vi "BRig_Host__Loop_Producer__UploadLaserParameters_main.vi"() -> ()   [LabVIEW 2014]
uses:
  <vilib>/WebDAVClient/NI_WebDAV.lvlib
panel:
  out "error out":errorcluster
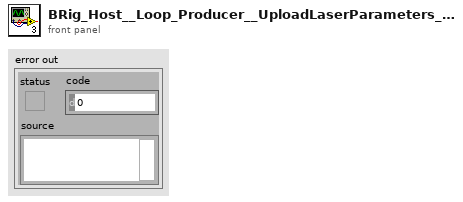
[diagram p1: front panel]
types:
  T1 = typedef "NI_WebDAV.lvlib/SessionHandle.ctl" = refnum<k1>
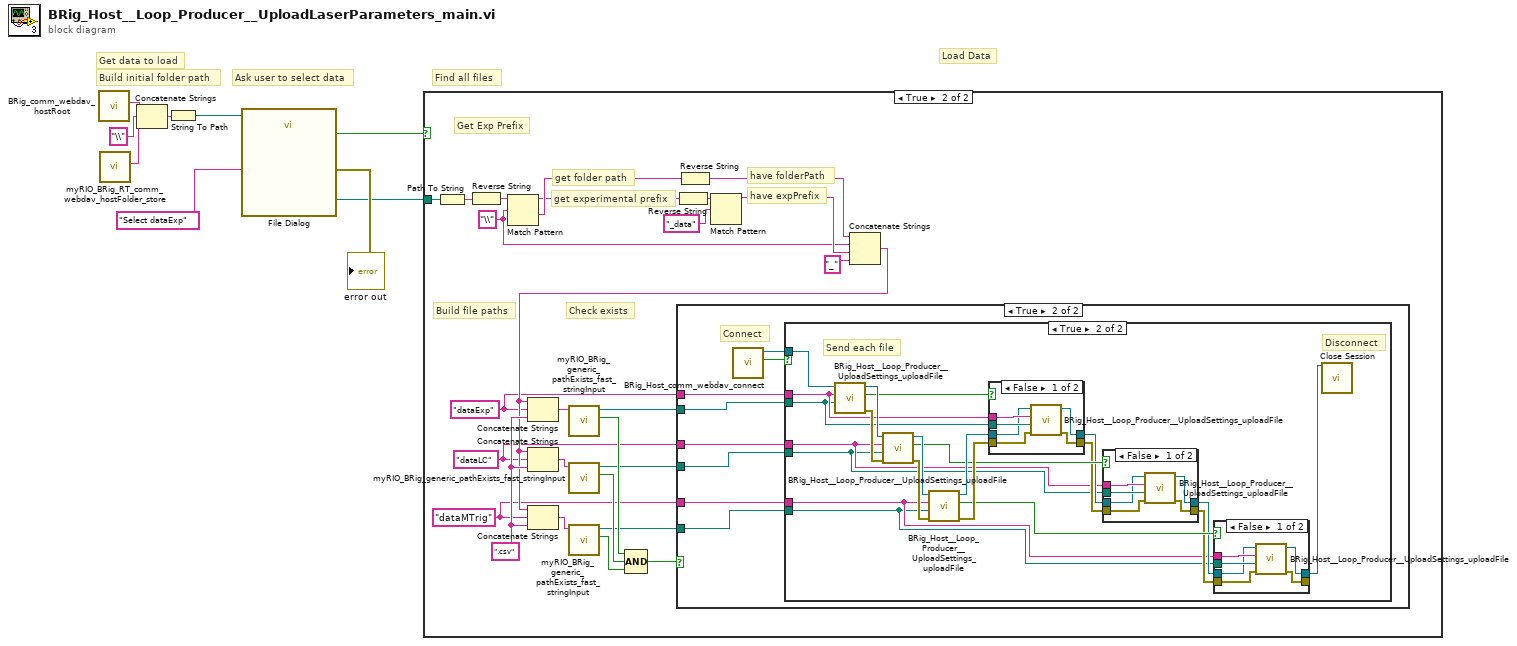
[diagram p0: block diagram]
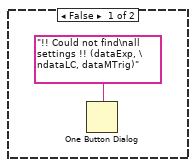
[diagram p3: hidden frame]
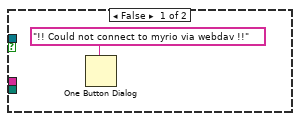
[diagram p4: hidden frame]
diagram:
  # "Load Data"
  # "Find all files"
  # "Ask user to select data"
  # "Build initial folder path"
  # "Get data to load"
  n1 = call "BRig_comm_webdav_hostRoot.vi"() -> ("output_hostRoot"=w6:string)  [unwired: 11 in]
  n2 = call "myRIO_BRig_RT_comm_webdav_hostFolder_store.vi"() -> ("output_HostFolder"=w8:string)  [unwired: 11 in]
  n3 = Concatenate Strings(w6, "\\" ("string"), w8) -> (w9:string)
  n4 = String To Path(string=w9) -> (path=w5:path)
  n5 = call "File Dialog"("start path"=w5, "prompt"="Select dataExp") -> ("selected path"=w1:path, "exists"=w2:bool, "error out"=→"error out":errorcluster)  [unwired: 10 in, 1 out]
  n6 = case shown="True" w2 {
    tunnel: w1 -> [_ w25]
    frame False {
    }
    frame True {
      w10 = "dataMTrig" ("regular expression")
      w11 = "dataLC" ("regular expression")
      w24 = ".csv" ("string")
      w12 = "dataExp" ("regular expression")
      w33 = "\\" ("regular expression")
      # "Check exists"
      # "Build file paths"
      # "get folder path"
      # "get experimental prefix"
      # "have expPrefix"
      # "have folderPath"
      # "Get Exp Prefix"
      n7 = Path To String(path=w25) -> (string=w26:string)
      n8 = Reverse String(1:w26) -> (0:w27:string)
      n9 = Match Pattern(string=w27, regular expression=w33) -> (before substring=w28:string, after substring=w31:string)  [unwired: 1 in, 2 out]
      n10 = Reverse String(1:w28) -> (0:w29:string)
      n11 = Reverse String(1:w31) -> (0:w32:string)
      n12 = Match Pattern(string=w29, regular expression="_data") -> (before substring=w34:string)  [unwired: 1 in, 3 out]
      n13 = Concatenate Strings(w32, w33, w34, "_" ("string")) -> (w23:string)
      n14 = Concatenate Strings(w23, w12, w24) -> (w22:string)
      n15 = Concatenate Strings(w23, w11, w24) -> (w21:string)
      n16 = Concatenate Strings(w23, w10, w24) -> (w20:string)
      n17 = call "myRIO_BRig_generic_pathExists_fast_stringInput.vi"("input_filePath"=w22) -> ("output_Iexist"=w19:bool, "output_filePath"=w15:path)  [unwired: 8 in, 1 out]
      n18 = call "myRIO_BRig_generic_pathExists_fast_stringInput.vi"("input_filePath"=w21) -> ("output_Iexist"=w18:bool, "output_filePath"=w14:path)  [unwired: 8 in, 1 out]
      n19 = call "myRIO_BRig_generic_pathExists_fast_stringInput.vi"("input_filePath"=w20) -> ("output_Iexist"=w17:bool, "output_filePath"=w13:path)  [unwired: 8 in, 1 out]
      n20 = Compound Arithmetic op=AND(w19, w18, w17) -> (w16:bool)
      n21 = case shown="True" w16 {
        tunnel: w15 -> [_ w42]
        tunnel: w14 -> [_ w39]
        tunnel: w13 -> [_ w37]
        tunnel: w12 -> [_ w41]
        tunnel: w11 -> [_ w40]
        tunnel: w10 -> [_ w38]
        frame False {
          n22 = One Button Dialog(message="!! Could not find\nall settings !! (dataExp, \ndataLC, dataMTrig)") -> ()  [unwired: 1 in, 1 out]
        }
        frame True {
          # "Connect"
          n23 = call "BRig_Host_comm_webdav_connect.vi"() -> ("output_Iconnected"=w44:bool, "output_hSession"=w43:T1)  [unwired: 9 in, 1 out]
          n24 = case shown="True" w44 {
            tunnel: w43 -> [_ w66]
            tunnel: w42 -> [_ w59]
            tunnel: w41 -> [_ w60]
            tunnel: w40 -> [_ w53]
            tunnel: w39 -> [_ w52]
            tunnel: w38 -> [_ w48]
            tunnel: w37 -> [_ w47]
            frame False {
              n25 = One Button Dialog(message="!! Could not connect to myrio via webdav !!") -> ()  [unwired: 1 in, 1 out]
            }
            frame True {
              # "Send each file"
              # "Disconnect"
              n26 = call "BRig_Host__Loop_Producer__UploadSettings_uploadFile.vi"("input_filePath_local"=w59, "dataName"=w60, "input_hSession"=w66) -> ("output_error"=w64:errorcluster, "output_Iexist"=w61:bool, "output_hSession"=w65:T1)  [unwired: 6 in]
              n27 = call "BRig_Host__Loop_Producer__UploadSettings_uploadFile.vi"("input_error"=w64, "input_filePath_local"=w52, "dataName"=w53, "input_hSession"=w65) -> ("output_error"=w62:errorcluster, "output_Iexist"=w56:bool, "output_hSession"=w63:T1)  [unwired: 5 in]
              n28 = call "BRig_Host__Loop_Producer__UploadSettings_uploadFile.vi"("input_error"=w62, "input_filePath_local"=w47, "dataName"=w48, "input_hSession"=w63) -> ("output_error"=w57:errorcluster, "output_Iexist"=w51:bool, "output_hSession"=w58:T1)  [unwired: 5 in]
              n29 = case shown="False" w61 {
                tunnel: w60 -> [w88 _]
                tunnel: w59 -> [w87 _]
                tunnel: w58 -> [w86 w90]
                tunnel: w57 -> [w85 w89]
                tunnel: [w84 w90] -> w55
                tunnel: [w83 w89] -> w54
                frame False {
                  n30 = call "BRig_Host__Loop_Producer__UploadSettings_uploadFile.vi"("input_error"=w85, "input_filePath_local"=w87, "dataName"=w88, "input_hSession"=w86) -> ("output_error"=w83:errorcluster, "output_hSession"=w84:T1)  [unwired: 5 in, 1 out]
                }
                frame True {
                }
              }
              n31 = case shown="False" w56 {
                tunnel: w53 -> [w80 _]
                tunnel: w52 -> [w79 _]
                tunnel: w55 -> [w78 w82]
                tunnel: w54 -> [w77 w81]
                tunnel: [w76 w82] -> w50
                tunnel: [w75 w81] -> w49
                frame False {
                  n32 = call "BRig_Host__Loop_Producer__UploadSettings_uploadFile.vi"("input_error"=w77, "input_filePath_local"=w79, "dataName"=w80, "input_hSession"=w78) -> ("output_error"=w75:errorcluster, "output_hSession"=w76:T1)  [unwired: 5 in, 1 out]
                }
                frame True {
                }
              }
              n33 = case shown="False" w51 {
                tunnel: w48 -> [w72 _]
                tunnel: w47 -> [w71 _]
                tunnel: w50 -> [w70 w74]
                tunnel: w49 -> [w69 w73]
                tunnel: [w68 w74] -> w46
                tunnel: [w67 w73] -> _
                frame False {
                  n34 = call "BRig_Host__Loop_Producer__UploadSettings_uploadFile.vi"("input_error"=w69, "input_filePath_local"=w71, "dataName"=w72, "input_hSession"=w70) -> ("output_error"=w67:errorcluster, "output_hSession"=w68:T1)  [unwired: 5 in, 1 out]
                }
                frame True {
                }
              }
              n35 = call <vilib>:"Close Session.vi"("session handle"=w46) -> ()  [unwired: 14 in, 1 out]
            }
          }
        }
      }
    }
  }
